vi "Define BC.vi"(5 "target BC":refnum<class "NI_BC.lvclass">, 6 "index":i32, 7 "target PDE":refnum<class "NI_PDE.lvclass">, 8 "error in (no error)":errorcluster, 10 "BC":variant, 11 "PDE in":refnum<class "NI_PDE.lvclass">) -> (0 "error out":errorcluster, 3 "PDE out":refnum<class "NI_PDE.lvclass">)   [LabVIEW 2020, in "NI_PDE.lvlib" / "NI_PDE.lvclass"]
uses:
  <vilib>/gmath/pde.llb/PDEClass/NI_PDE.lvclass
  <vilib>/gmath/pde.llb/BCClass/NI_BC.lvclass
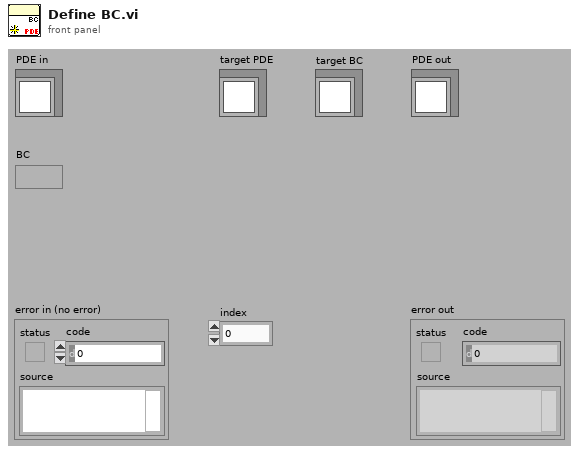
[diagram p1: front panel]
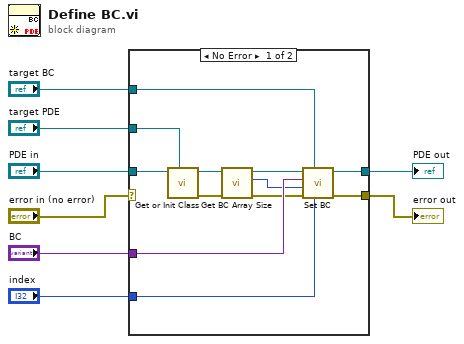
[diagram p0: block diagram]
diagram:
  n1 = case shown="No Error" "error in (no error)" {
    selector: "error in (no error)" -> [_ w22]
    tunnel: "PDE in" -> [w17 w21]
    tunnel: [w20 w21] -> w8
    tunnel: [w19 w22] -> w7
    tunnel: "target BC" -> [w14 _]
    tunnel: "target PDE" -> [w15 _]
    tunnel: "BC" -> [w18 _]
    tunnel: "index" -> [w16 _]
    frame No Error {
      n2 = call <vilib>:"Get or Init Class.vi"("target PDE"=w15, "PDE in"=w17) -> ("error out"=w12:errorcluster, "PDE out"=w13:refnum<class "NI_PDE.lvclass">)  [unwired: 2 in, 6 out]
      n3 = call-dynamic "Get BC Array Size.vi"("error in (no error)"=w12, "PDE in"=w13) -> ("error out"=w10:errorcluster, "# of BC"=w9:i32, "PDE out"=w11:refnum<class "NI_PDE.lvclass">)  [unwired: 7 out]
      n4 = call <vilib>:"Set BC.vi"("index"=w16, "target BC"=w14, "error in (no error)"=w10, "# of BC"=w9, "BC"=w18, "PDE in"=w11) -> ("error out"=w19:errorcluster, "PDE out"=w20:refnum<class "NI_PDE.lvclass">)  [unwired: 4 out]
    }
    frame Error {
    }
  }
  "PDE out" <- w8
  "error out" <- w7
